vi "Pyht.vi"(1 "B":dbl, 2 "A":dbl) -> (0 "C":dbl)   [LabVIEW 2019]
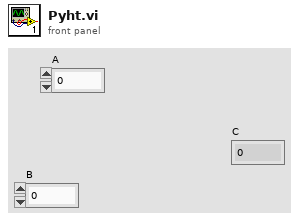
[diagram p1: front panel]
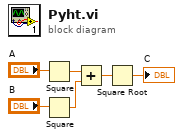
[diagram p0: block diagram]
diagram:
  n1 = Square(x="A") -> (x^2=w4:dbl)
  n2 = Square(x="B") -> (x^2=w3:dbl)
  n3 = Add(x=w4, y=w3) -> (x+y=w2:dbl)
  n4 = Square Root(x=w2) -> (sqrt(x)=→"C":dbl)
